vi "initIP.vi"() -> ()   [LabVIEW 2010]
uses:
  AmmeterGlobalCostants.vi
panel:
  in  "PortIPList 2":string[](array[string])=["700443111200", "690443111200", "710443111200", "680443111200"]
  in  "PortIPList":string[](array[string])=["040000000000", "030000000000", "010000000000", "020000000000"]
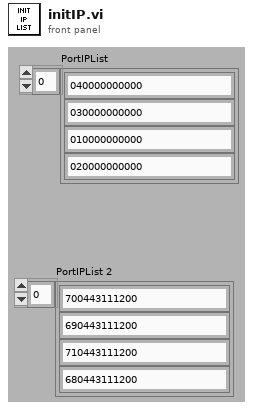
[diagram p1: front panel]
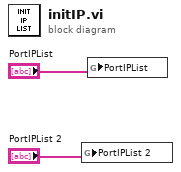
[diagram p0: block diagram]
diagram:
  n1 = global write "AmmeterGlobalCostants.vi" "PortIPList 2"("PortIPList 2") -> ()
  n2 = global write "AmmeterGlobalCostants.vi" "PortIPList"("PortIPList") -> ()
